vi "Read Owner Event Ref.vi"(8 "error in (no error)":errorcluster, 11 "Attribute.Owner in":refnum<class "Attribute.Owner.lvclass">) -> (0 "error out":errorcluster, 2 "Upstream Ref":refnum<user-event>, 3 "Attribute.Owner out":refnum<class "Attribute.Owner.lvclass">)   [LabVIEW 2021, in "smo.lvlib" / "Attribute.Owner.lvclass"]
uses:
  Attribute.Owner.lvclass
  Packet -- Cluster.ctl
  Attribute.Owner.lvclass/Attribute.Owner.ctl
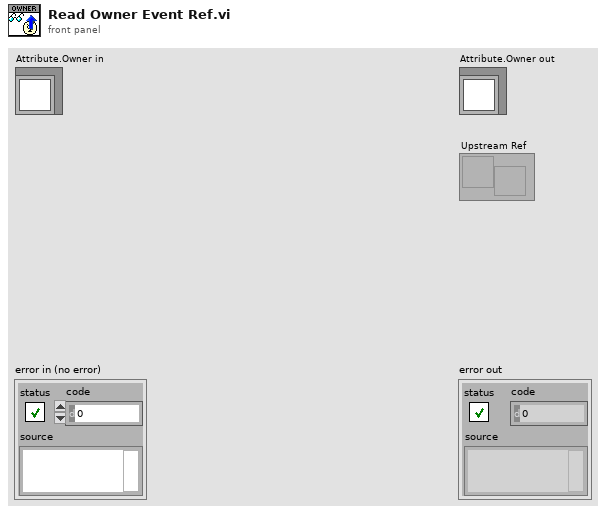
[diagram p1: front panel]
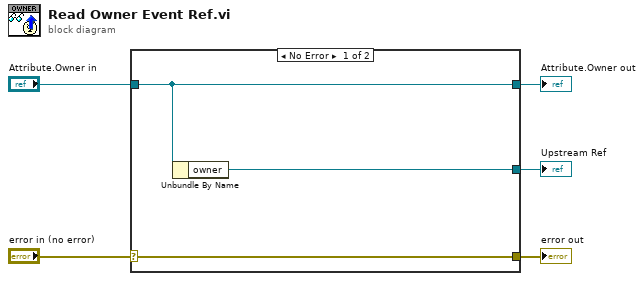
[diagram p0: block diagram]
diagram:
  n1 = case shown="No Error" "error in (no error)" {
    selector: "error in (no error)" -> [w8 w9]
    tunnel: [w8 w9] -> w4
    tunnel: [w7 w10] -> w2
    tunnel: "Attribute.Owner in" -> [w7 w10]
    tunnel: [w6 _] -> w1
    frame No Error {
      n2 = Unbundle By Name(w7) -> ("owner"=w6:refnum<user-event>)
    }
    frame Error {
    }
  }
  "error out" <- w4
  "Attribute.Owner out" <- w2
  "Upstream Ref" <- w1
